vi "GET_engine_data.vi"(8 "API Key":string="cheia04042025tema2restfulapi") -> (0 "engine info":T1, 1 "body":string, 2 "headers":string)   [LabVIEW 2024]
uses:
  <vilib>/httpClient/LabVIEWHTTPClient.lvlib
panel:
  out "error out json":errorcluster
  out "error out get":errorcluster
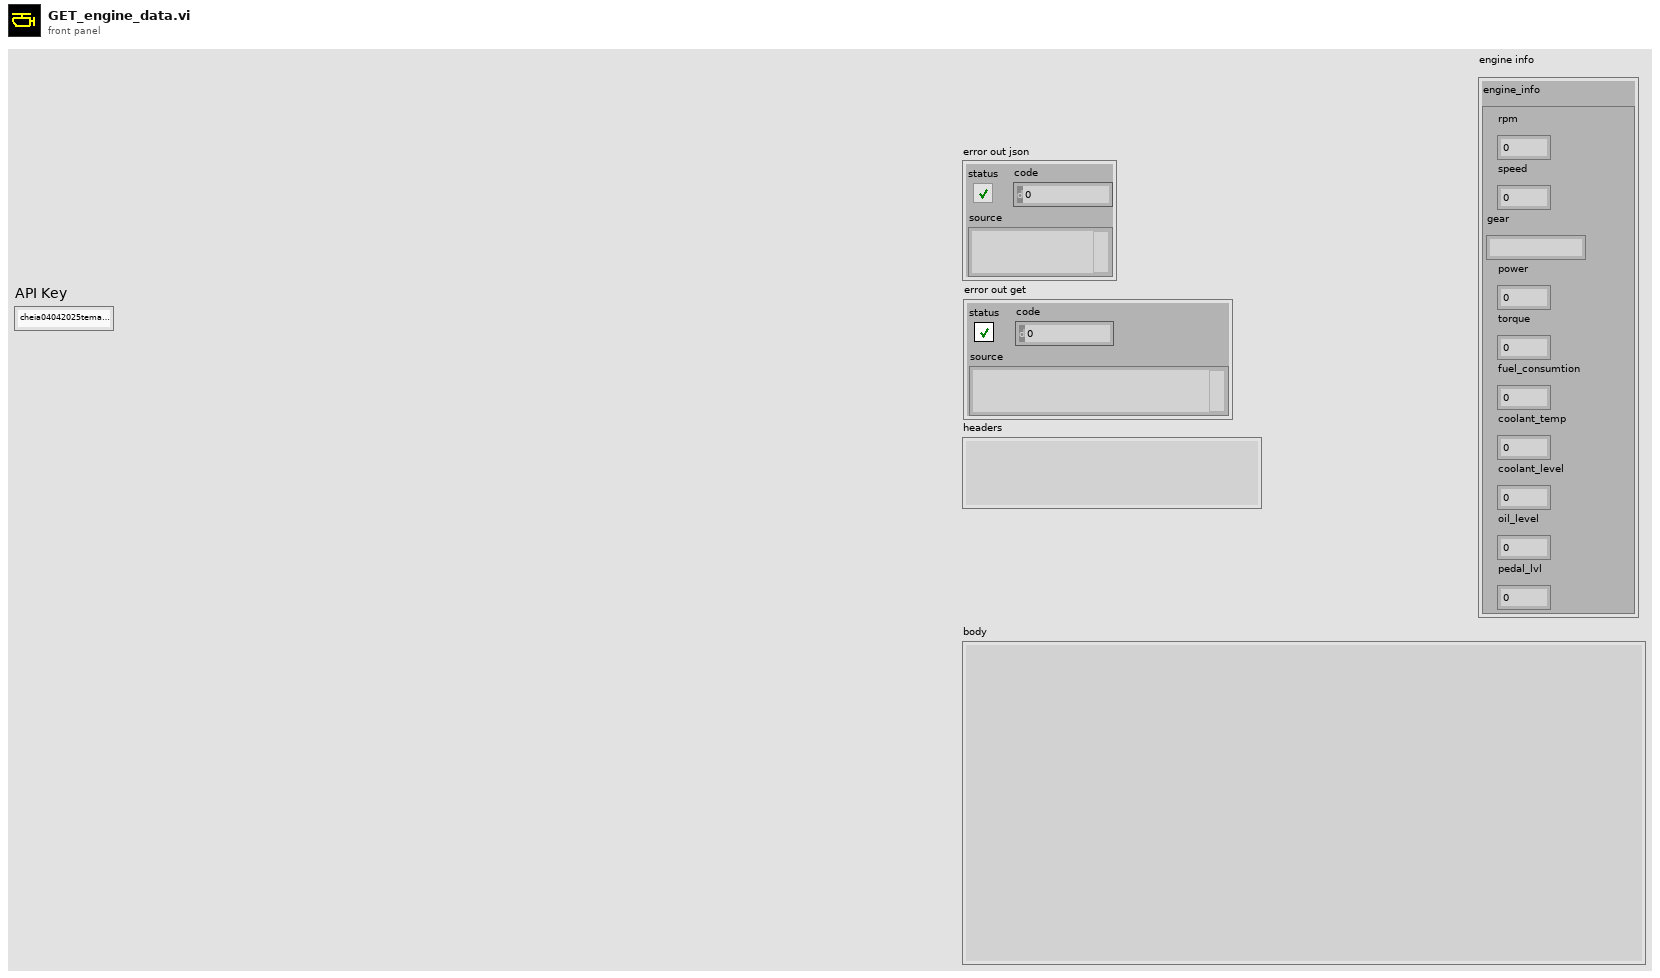
[diagram p1: front panel]
types:
  T1 = cluster{"engine_info":cluster{"rpm":u64, "speed":u64, "gear":string, "power":i32, "torque":i32, "fuel_consumtion":dbl, "coolant_temp":i32, "coolant_level":i32, "oil_level":i32, "pedal_lvl":i32}}
  T2 = typedef "LabVIEWHTTPClient.lvlib/ClientHandle.ctl" = refnum<k1>
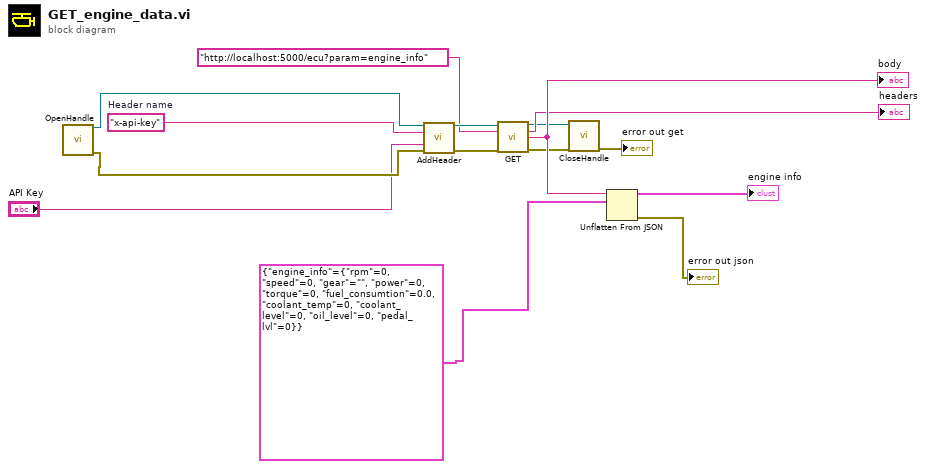
[diagram p0: block diagram]
diagram:
  w5 = "x-api-key"  # Header name
  n1 = call <vilib>:"OpenHandle.vi"() -> ("client handle out"=w6:T2, "error out"=w7:errorcluster)  [unwired: 14 in]
  n2 = call <vilib>:"AddHeader.vi"("client handle"=w6, "header"=w5, "value"="API Key", "error in (no error)"=w7) -> ("client handle out"=w9:T2, "error out"=w8:errorcluster)  [unwired: 10 in]
  n3 = call <vilib>:"GET.vi"("client handle"=w9, "url"="http://localhost:5000/ecu?param=engine_info", "error in (no error)"=w8) -> ("client handle out"=w11:T2, "headers"=→"headers":string, "body"=w15:string, "error out"=w10:errorcluster)  [unwired: 9 in]
  "body" <- w15
  n4 = call <vilib>:"CloseHandle.vi"("client handle"=w11, "error in (no error)"=w10) -> ("error out"=→"error out get":errorcluster)  [unwired: 13 in]
  n5 = Unflatten From JSON(JSON string=w15, type and defaults=T1 {"engine_info"={"rpm"=0, "speed"=0, "gear"="", "power"=0, "torque"=0, "fuel_consumtion"=0.0, "coolant_temp"=0, "coolant_level"=0, "oil_level"=0, "pedal_lvl"=0}}) -> (value=→"engine info":T1, error out=→"error out json":errorcluster)  [unwired: 5 in]
